vi "get connected terminals.vi"(8 "error in":errorcluster, 10 "all terms":refnum<vi>[](array[refnum]), 11 "excluded term":refnum<vi>) -> (0 "error out":errorcluster, 3 "other terms":refnum<vi>[](array[refnum]))   [LabVIEW 2013, in "DecideModuleFeatures.lvclass"]
uses:
  DecideModuleFeatures.lvclass
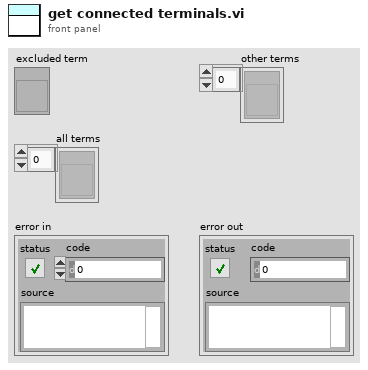
[diagram p1: front panel]
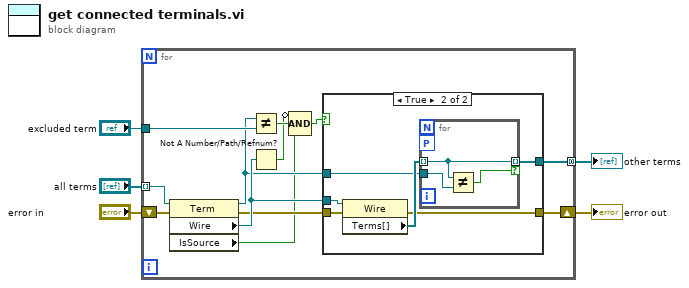
[diagram p0: block diagram]
diagram:
  n1 = for {
    tunnel: "all terms" -> [w17] mode=indexing
    tunnel: "excluded term" -> [w16]
    shift-right: [w10] -> w2
    shift-left: "error in" -> [w15]
    tunnel: [w7] -> w1 mode=concatenating
    n2 = property class="Term"(reference=w17, error in=w15) -> (reference out=w8:refnum<vi>, error out=w9:errorcluster, "Wire"=w11:refnum<vi>, "IsSource"=w6:bool)
    n3 = Not Equal?(x=w8, y=w16) -> (x != y?=w14:bool)
    n4 = Not A Number/Path/Refnum?(number/path/refnum=w11) -> (NaN/Path/Refnum?=w13:bool)
    n5 = Compound Arithmetic op=AND(invert w13, w14, w6) -> (w12:bool)
    n6 = case shown="True" w12 {
      tunnel: w11 -> [_ w24]
      tunnel: [w18 w19] -> w10
      tunnel: w9 -> [w18 w23]
      tunnel: w8 -> [_ w21]
      tunnel: [_ w20] -> w7
      frame False {
      }
      frame True {
        n7 = property class="Wire"(reference=w24, error in=w23) -> (error out=w19:errorcluster, "Terms[]"=w22:refnum<vi>[])  [unwired: 1 out]
        n8 = for {
          tunnel: w22 -> [w26] mode=indexing
          tunnel: w21 -> [w27]
          tunnel: [w26] -> w20 mode=indexing if=w25
          workers-P: _ -> [_]
          n9 = Not Equal?(x=w26, y=w27) -> (x != y?=w25:bool)
        }
      }
    }
  }
  "error out" <- w2
  "other terms" <- w1
